vi "参数解析.vi"(10 "指令格式":string[](array[string]), 11 "参数数组":u32[](array[numeric])) -> (3 "解析指令数组":string[](array[string]))   [LabVIEW 2016]
panel:
  out "指令状态":string
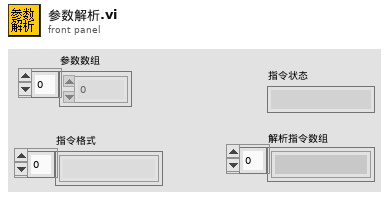
[diagram p1: front panel]
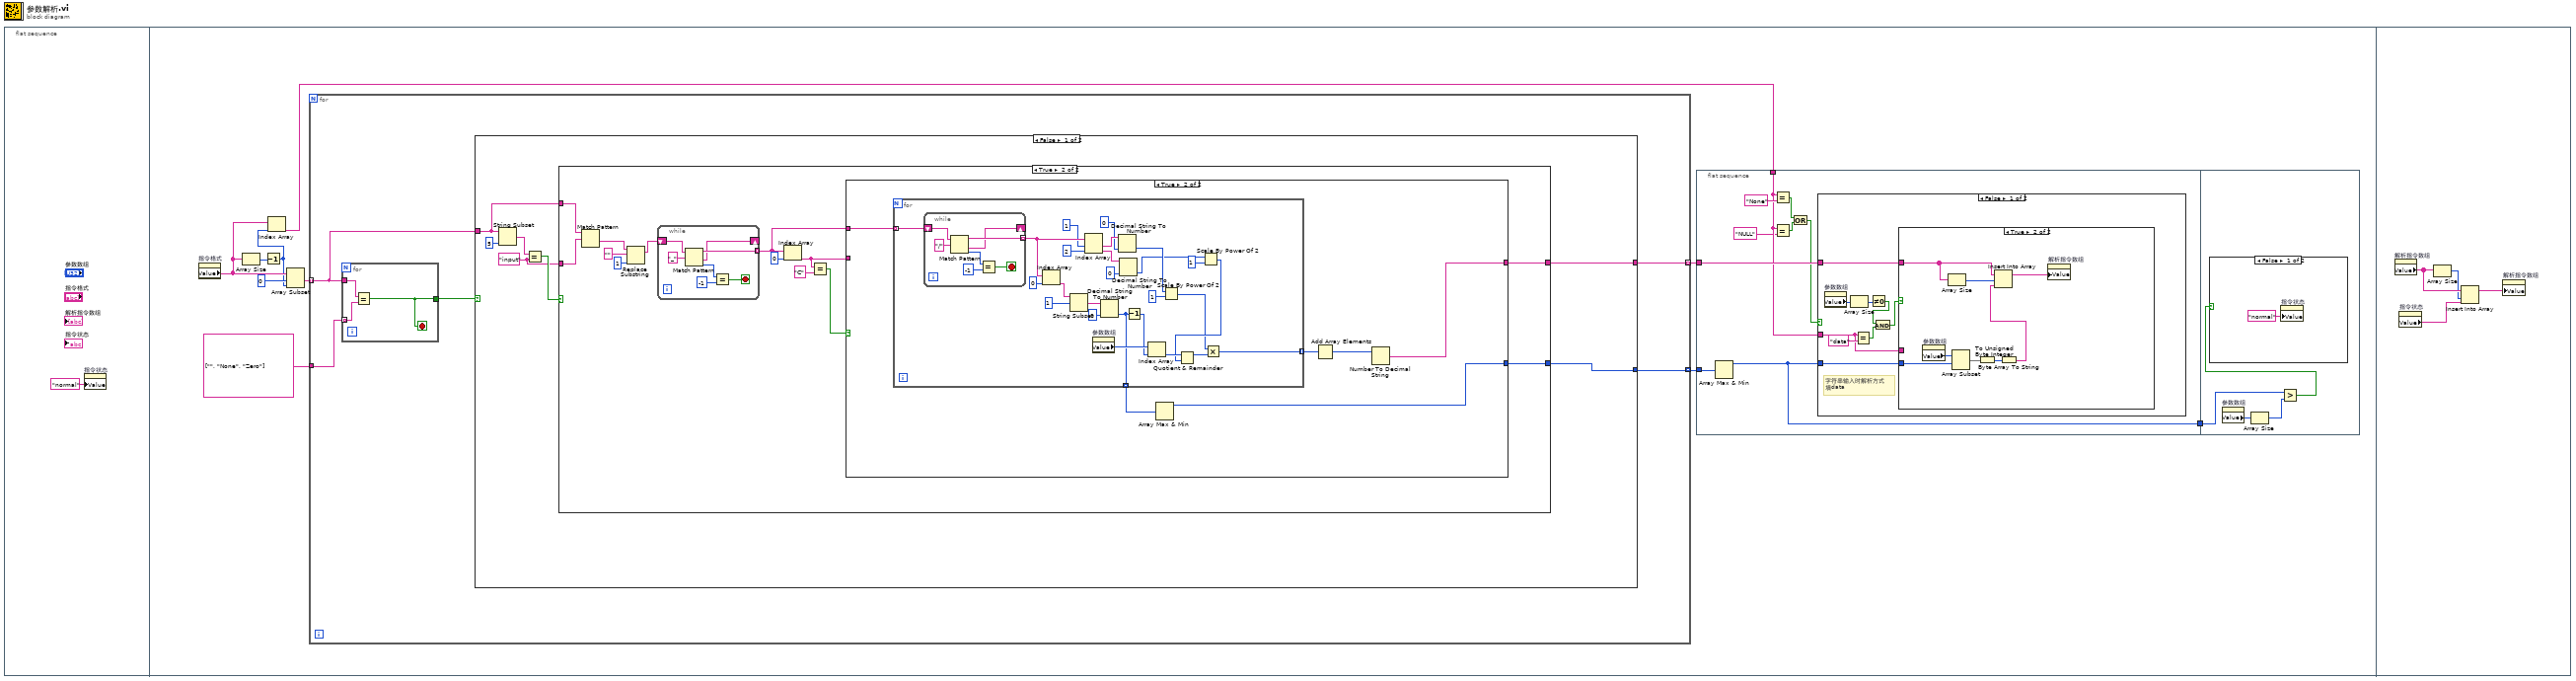
[diagram p0: block diagram]
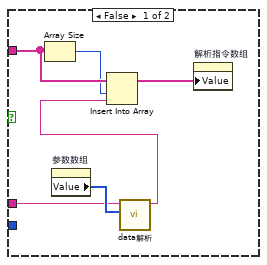
[diagram p2: hidden frame]
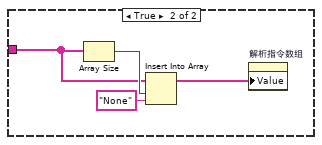
[diagram p3: hidden frame]
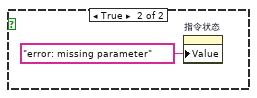
[diagram p4: hidden frame]
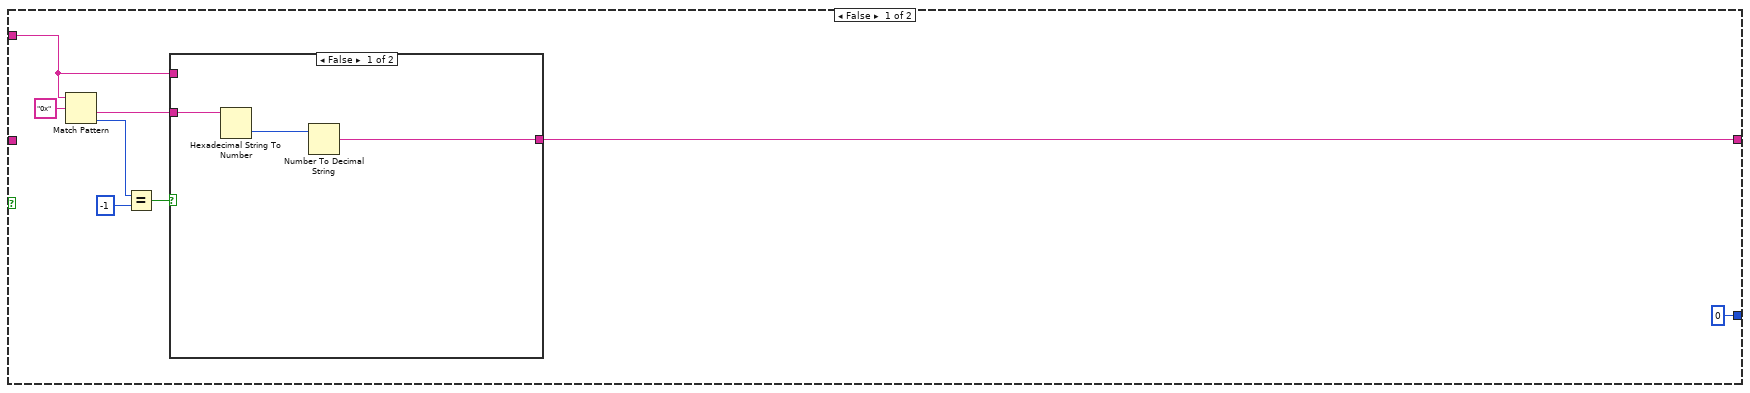
[diagram p5: hidden frame]
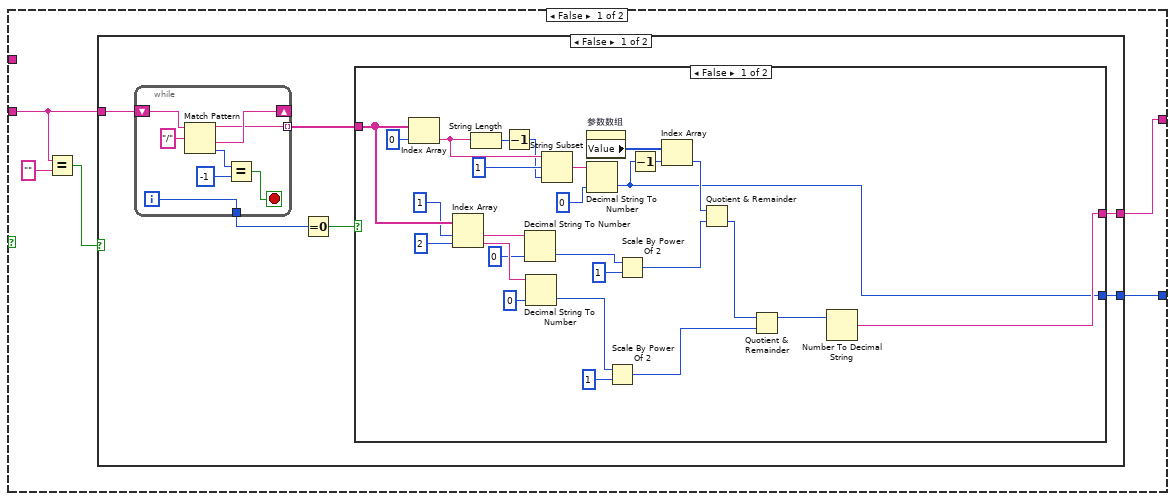
[diagram p7: hidden frame]
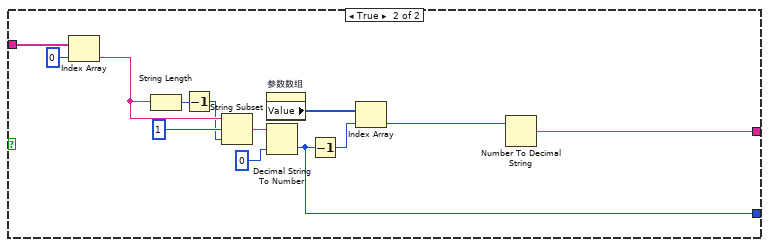
[diagram p8: hidden frame]
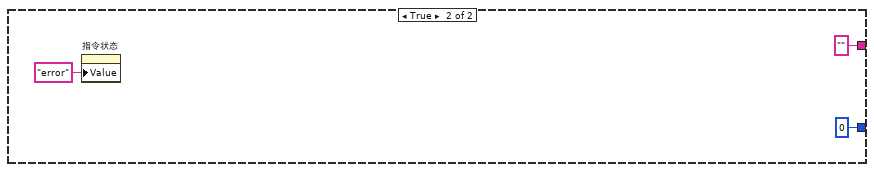
[diagram p9: hidden frame]
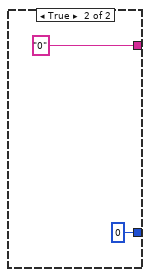
[diagram p10: hidden frame]
diagram:
  n1 = flat-sequence {
    frame #0 {
      n2 = property on="指令状态" class="Str"("Value"="normal" ("指令状态")) -> ()  [unwired: 2 in, 2 out]
    }
    frame #1 {
      n3 = property on="指令格式" class="Arr (strict)"() -> ("Value"=w7:string[])  [unwired: 2 in, 2 out]
      n4 = Array Size(array=w7) -> (size(s)=w8:i32)
      n5 = Decrement(x=w8) -> (x-1=w6:i32)
      n6 = Index Array(array=w7, index=w6) -> (element=w3:string)
      n7 = Array Subset(array=w7, index=0 ("索引"), length=w6) -> (w10:string[])
      n8 = for {
        tunnel: w10 -> [w56] mode=indexing
        tunnel: string[] ["", "None", "Zero"] -> [w58]
        tunnel: [w55] -> w4 mode=indexing
        tunnel: [w54] -> w5 mode=indexing
        n9 = for {
          tunnel: w56 -> [w202]
          tunnel: w58 -> [w201] mode=indexing
          tunnel: [w200] -> w57
          stop <- w200 stop-if-true
          n10 = Equal?(x=w202, y=w201) -> (x = y?=w200:bool)
        }
        n11 = case shown="False" w57 {
          tunnel: [w60 "0"] -> w55
          tunnel: w56 -> [w62 _]
          tunnel: [w59 u32 0] -> w54
          frame False {
            w61 = "input" ("y")
            n12 = String Subset(string=w62, length (rest)=5 ("长度（剩余）")) -> (substring=w64:string)  [unwired: 1 in]
            n13 = Equal?(x=w64, y=w61) -> (x = y?=w63:bool)
            n14 = case shown="True" w63 {
              tunnel: w62 -> [w67 w90]
              tunnel: [w68 w80] -> w60
              tunnel: w61 -> [_ w89]
              tunnel: [u32 0 w78] -> w59
              frame False {
                n15 = Match Pattern(string=w67, regular expression="0x" ("正则表达式")) -> (after substring=w69:string, offset past match=w71:i32)  [unwired: 1 in, 2 out]
                n16 = Equal?(x=w71, y=-1) -> (x = y?=w72:bool)
                n17 = case shown="False" w72 {
                  tunnel: w69 -> [w76 _]
                  tunnel: [w74 w77] -> w68
                  tunnel: w67 -> [_ w77]
                  frame False {
                    n18 = Hexadecimal String To Number(string=w76) -> (number=w75:u32)  [unwired: 2 in, 1 out]
                    n19 = Number To Decimal String(number=w75) -> (decimal integer string=w74:string)  [unwired: 1 in]
                  }
                  frame True {
                  }
                }
              }
              frame True {
                n20 = Match Pattern(string=w90, regular expression=w89) -> (after substring=w86:string)  [unwired: 1 in, 3 out]
                n21 = Replace Substring(2:1 ("长度（子字符串长度）"), 4:"" ("子字符串(\"\")"), 5:w86) -> (1:w85:string)  [unwired: 1 in, 1 out]
                n22 = while {
                  tunnel: [w192] -> w81 mode=indexing
                  shift-right: [w191] -> _
                  shift-left: w85 -> [w197]
                  stop <- w193 stop-if-true
                  n23 = Match Pattern(string=w197, regular expression="_" ("正则表达式")) -> (before substring=w192:string, after substring=w191:string, offset past match=w195:i32)  [unwired: 1 in, 1 out]
                  n24 = Equal?(x=w195, y=-1) -> (x = y?=w193:bool)
                }
                n25 = Index Array(array=w81, index=0 ("索引")) -> (element=w79:string)
                n26 = Equal?(x=w79, y="C") -> (x = y?=w82:bool)
                n27 = case shown="True" w82 {
                  tunnel: w81 -> [_ w158]
                  tunnel: [w92 w155] -> w80
                  tunnel: w79 -> [w95 _]
                  tunnel: [w91 w153] -> w78
                  frame False {
                    n28 = Equal?(x=w95, y="") -> (x = y?=w93:bool)
                    n29 = case shown="False" w93 {
                      tunnel: w95 -> [w100 _]
                      tunnel: [w97 ""] -> w92
                      tunnel: [w96 0] -> w91
                      frame False {
                        n30 = while {
                          shift-right: [w148] -> _
                          shift-left: w100 -> [w149]
                          tunnel: [w144] -> w101
                          tunnel: [w142] -> w98 mode=indexing
                          i -> [w144]
                          stop <- w145 stop-if-true
                          n31 = Match Pattern(string=w149, regular expression="/" ("正则表达式")) -> (before substring=w142:string, after substring=w148:string, offset past match=w147:i32)  [unwired: 1 in, 1 out]
                          n32 = Equal?(x=w147, y=-1) -> (x = y?=w145:bool)
                        }
                        n33 = Equal To 0?(x=w101) -> (x = 0?=w99:bool)
                        n34 = case shown="False" w99 {
                          tunnel: w98 -> [w121 w141]
                          tunnel: [w107 w134] -> w97
                          tunnel: [w105 w130] -> w96
                          frame False {
                            n35 = Index Array(array=w121, index=0 ("索引")) -> (element=w126:string)
                            n36 = Index Array(array=w121, index #1=1 ("索引"), index #2=2 ("索引")) -> (element #1=w118:string, element #2=w117:string)
                            n37 = String Length(string=w126) -> (length=w125:i32)
                            n38 = Decrement(x=w125) -> (x-1=w124:i32)
                            n39 = Decimal String To Number(string=w118, default (0L)=u32 0 ("默认(0 I32)")) -> (number=w115:u32)  [unwired: 1 in, 1 out]
                            n40 = Decimal String To Number(string=w117, default (0L)=u32 0 ("默认(0 I32)")) -> (number=w113:u32)  [unwired: 1 in, 1 out]
                            n41 = String Subset(string=w126, offset (0)=1 ("偏移量(0)"), length (rest)=w124) -> (substring=w123:string)
                            n42 = property on="参数数组" class="Arr (strict)"() -> ("Value"=w122:u32[])  [unwired: 2 in, 2 out]
                            n43 = Decimal String To Number(string=w123, default (0L)=u32 0 ("默认(0 I32)")) -> (number=w105:u32)  [unwired: 1 in, 1 out]
                            n44 = Scale By Power Of 2(n=w113, x=u32 1) -> (x*2^n=w109:u32)
                            n45 = Scale By Power Of 2(n=w115, x=u32 1) -> (x*2^n=w111:u32)
                            n46 = Decrement(x=w105) -> (x-1=w106:u32)
                            n47 = Index Array(array=w122, index=w106) -> (element=w112:u32)
                            n48 = Quotient & Remainder(x=w112, y=w111) -> (floor(x/y)=w110:u32)  [unwired: 1 out]
                            n49 = Quotient & Remainder(x=w110, y=w109) -> (x-y*floor(x/y)=w108:u32)  [unwired: 1 out]
                            n50 = Number To Decimal String(number=w108) -> (decimal integer string=w107:string)  [unwired: 1 in]
                          }
                          frame True {
                            n51 = Index Array(array=w141, index=0 ("索引")) -> (element=w138:string)
                            n52 = String Length(string=w138) -> (length=w137:i32)
                            n53 = Decrement(x=w137) -> (x-1=w136:i32)
                            n54 = String Subset(string=w138, offset (0)=1 ("偏移量(0)"), length (rest)=w136) -> (substring=w135:string)
                            n55 = property on="参数数组" class="Arr (strict)"() -> ("Value"=w133:u32[])  [unwired: 2 in, 2 out]
                            n56 = Decimal String To Number(string=w135, default (0L)=u32 0 ("默认(0 I32)")) -> (number=w130:u32)  [unwired: 1 in, 1 out]
                            n57 = Decrement(x=w130) -> (x-1=w131:u32)
                            n58 = Index Array(array=w133, index=w131) -> (element=w132:u32)
                            n59 = Number To Decimal String(number=w132) -> (decimal integer string=w134:string)  [unwired: 1 in]
                          }
                        }
                      }
                      frame True {
                        n60 = property on="指令状态" class="Str"("Value"="error" ("指令状态")) -> ()  [unwired: 2 in, 2 out]
                      }
                    }
                  }
                  frame True {
                    n61 = for {
                      tunnel: w158 -> [w183] mode=indexing
                      tunnel: [w164] -> w157 mode=indexing
                      tunnel: [w162] -> w154 mode=indexing
                      n62 = while {
                        tunnel: [w185] -> w179 mode=indexing
                        shift-right: [w184] -> _
                        shift-left: w183 -> [w190]
                        stop <- w186 stop-if-true
                        n63 = Match Pattern(string=w190, regular expression="/" ("正则表达式")) -> (before substring=w185:string, after substring=w184:string, offset past match=w188:i32)  [unwired: 1 in, 1 out]
                        n64 = Equal?(x=w188, y=-1) -> (x = y?=w186:bool)
                      }
                      n65 = Index Array(array=w179, index=0 ("索引")) -> (element=w181:string)
                      n66 = String Subset(string=w181, offset (0)=1 ("偏移量(0)")) -> (substring=w176:string)  [unwired: 1 in]
                      n67 = Index Array(array=w179, index #1=1 ("索引"), index #2=2 ("索引")) -> (element #1=w175:string, element #2=w174:string)
                      n68 = property on="参数数组" class="Arr (strict)"() -> ("Value"=w173:u32[])  [unwired: 2 in, 2 out]
                      n69 = Decimal String To Number(string=w176, default (0L)=u32 0 ("默认(0 I32)")) -> (number=w162:u32)  [unwired: 1 in, 1 out]
                      n70 = Decimal String To Number(string=w175, default (0L)=u32 0 ("默认(0 I32)")) -> (number=w171:u32)  [unwired: 1 in, 1 out]
                      n71 = Decimal String To Number(string=w174, default (0L)=u32 0 ("默认(0 I32)")) -> (number=w169:u32)  [unwired: 1 in, 1 out]
                      n72 = Decrement(x=w162) -> (x-1=w163:u32)
                      n73 = Index Array(array=w173, index=w163) -> (element=w168:u32)
                      n74 = Scale By Power Of 2(n=w171, x=u32 1) -> (x*2^n=w166:u32)
                      n75 = Scale By Power Of 2(n=w169, x=u32 1) -> (x*2^n=w167:u32)
                      n76 = Quotient & Remainder(x=w168, y=w167) -> (x-y*floor(x/y)=w165:u32)  [unwired: 1 out]
                      n77 = Multiply(x=w166, y=w165) -> (x*y=w164:u32)
                    }
                    n78 = Array Max & Min(array=w154) -> (max value=w153:u32)  [unwired: 3 out]
                    n79 = Add Array Elements(numeric array=w157) -> (sum=w156:u32)
                    n80 = Number To Decimal String(number=w156) -> (decimal integer string=w155:string)  [unwired: 1 in]
                  }
                }
              }
            }
          }
          frame True {
          }
        }
      }
      n81 = flat-sequence {
        tunnel: w5 -> [w20]
        tunnel: w4 -> [w18]
        tunnel: w3 -> [w16]
        tunnel: [w17] -> w2
        tunnel: w2 -> [w49]
        frame #0 {
          n82 = Array Max & Min(array=w20) -> (max value=w17:u32)  [unwired: 3 out]
          n83 = Equal?(x=w16, y="None") -> (x = y?=w13:bool)
          n84 = Equal?(x=w16, y="NULL") -> (x = y?=w14:bool)
          n85 = Or(x=w13, y=w14) -> (x .or. y?=w12:bool)
          n86 = case shown="False" w12 {
            tunnel: w18 -> [w27 w45]
            tunnel: w17 -> [w26 _]
            tunnel: w16 -> [w21 _]
            frame False {
              # "字符串输入时解析方式\n填data"
              n87 = property on="参数数组" class="Arr (strict)"() -> ("Value"=w28:u32[])  [unwired: 2 in, 2 out]
              n88 = Array Size(array=w28) -> (size(s)=w29:i32)
              n89 = Equal?(x=w21, y="data") -> (x = y?=w23:bool)
              n90 = Not Equal To 0?(x=w29) -> (x != 0?=w24:bool)
              n91 = And(x=w24, y=w23) -> (x .and. y?=w22:bool)
              n92 = case shown="True" w22 {
                tunnel: w27 -> [w35 w37]
                tunnel: w26 -> [_ w42]
                tunnel: w21 -> [w31 _]
                frame False {
                  n93 = Array Size(array=w35) -> (size(s)=w34:i32)
                  n94 = property on="参数数组" class="Arr (strict)"() -> ("Value"=w32:u32[])  [unwired: 2 in, 2 out]
                  n95 = call "data解析.vi"("data_in"=w32, "格式字符串"=w31) -> ("输出字符串"=w30:string)  [unwired: 9 in]
                  n96 = Insert Into Array(array=w35, index=w34, new element=w30) -> (w33:string[])
                  n97 = property on="解析指令数组" class="Arr (strict)"("Value"=w33) -> ()  [unwired: 2 in, 2 out]
                }
                frame True {
                  n98 = property on="参数数组" class="Arr (strict)"() -> ("Value"=w43:u32[])  [unwired: 2 in, 2 out]
                  n99 = Array Size(array=w37) -> (size(s)=w36:i32)
                  n100 = Array Subset(array=w43, index=w42) -> (w41:u32[])  [unwired: 1 in]
                  n101 = To Unsigned Byte Integer(number=w41) -> (unsigned 8bit integer=w40:u8[])
                  n102 = Byte Array To String(unsigned byte array=w40) -> (string=w39:string)
                  n103 = Insert Into Array(array=w37, index=w36, new element=w39) -> (w38:string[])
                  n104 = property on="解析指令数组" class="Arr (strict)"("Value"=w38) -> ()  [unwired: 2 in, 2 out]
                }
              }
            }
            frame True {
              n105 = Array Size(array=w45) -> (size(s)=w47:i32)
              n106 = Insert Into Array(array=w45, index=w47, new element="None" ("新元素/子数组")) -> (w44:string[])
              n107 = property on="解析指令数组" class="Arr (strict)"("Value"=w44) -> ()  [unwired: 2 in, 2 out]
            }
          }
        }
        frame #1 {
          n108 = property on="参数数组" class="Arr (strict)"() -> ("Value"=w50:u32[])  [unwired: 2 in, 2 out]
          n109 = Array Size(array=w50) -> (size(s)=w51:i32)
          n110 = Greater?(x=w49, y=w51) -> (0:w48:bool)
          n111 = case shown="False" w48 {
            frame False {
              n112 = property on="指令状态" class="Str"("Value"="normal" ("指令状态")) -> ()  [unwired: 2 in, 2 out]
            }
            frame True {
              n113 = property on="指令状态" class="Str"("Value"="error: missing parameter" ("指令状态")) -> ()  [unwired: 2 in, 2 out]
            }
          }
        }
      }
    }
    frame #2 {
      n114 = property on="解析指令数组" class="Arr (strict)"() -> ("Value"=w206:string[])  [unwired: 2 in, 2 out]
      n115 = property on="指令状态" class="Str"() -> ("Value"=w204:string)  [unwired: 2 in, 2 out]
      n116 = Array Size(array=w206) -> (size(s)=w205:i32)
      n117 = Insert Into Array(array=w206, index=w205, new element=w204) -> (w203:string[])
      n118 = property on="解析指令数组" class="Arr (strict)"("Value"=w203) -> ()  [unwired: 2 in, 2 out]
    }
  }
